vi "RemoveDuplicates_2DArray.vi"(11 "Input Array":string[][](array[string])) -> (3 "Removed Duplicate Array":string[][](array[string]))   [LabVIEW 2020]
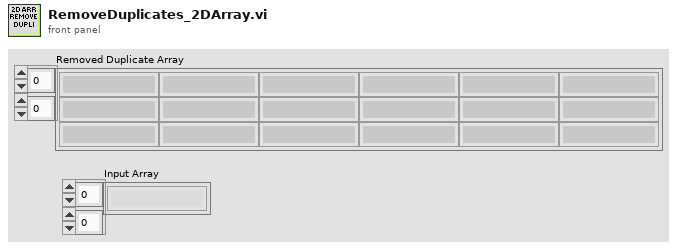
[diagram p1: front panel]
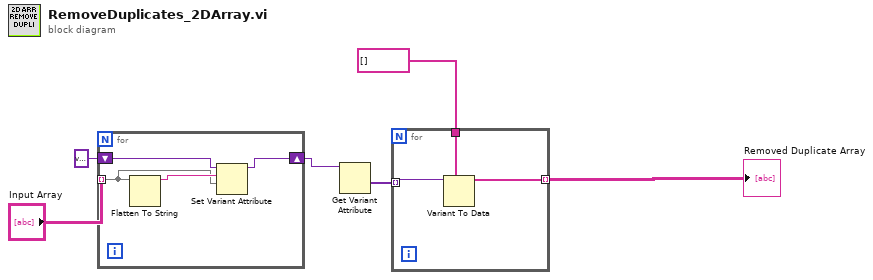
[diagram p0: block diagram]
diagram:
  n1 = for {
    tunnel: "Input Array" -> [w9] mode=indexing
    shift-right: [w7] -> w3
    shift-left: variant -> [w8]
    n2 = Flatten To String(anything=w9) -> (data string=w10:string)  [unwired: 3 in, 2 out]
    n3 = Set Variant Attribute(Variant=w8, name=w10, value=w9) -> (Variant out=w7:variant)  [unwired: 1 in, 2 out]
  }
  n4 = Get Variant Attribute(Variant=w3) -> (values=w4:variant[])  [unwired: 3 in, 3 out]
  n5 = for {
    tunnel: w4 -> [w13] mode=indexing
    tunnel: string[] [] ("Item Names") -> [w12]
    tunnel: [w11] -> w6 mode=indexing
    n6 = Variant To Data(type=w12, Variant=w13) -> (data=w11:string[])  [unwired: 1 in, 1 out]
  }
  "Removed Duplicate Array" <- w6
